vi "Read Channels.vi"(11 "HW Inline Ctrl in":T1 {"Input Channels"."Input Block Data Refs"."Data Reference" format="%.0x"; "Output Channels"."Output Block Data Refs"."Data Reference" format="%.0x"}) -> (3 "HW Inline Ctrl out":T1 {"Input Channels"."Input Block Data Refs"."Data Reference" format="%.0x"; "Output Channels"."Output Block Data Refs"."Data Reference" format="%.0x"})   [LabVIEW 2012, in "Shared Variable Custom Device.lvlib"]
doc: "Reads the values from the Input Block Data References and writes the values to the RT FIFO Read."
uses:
  Shared Variable Custom Device.lvlib
  HW Inline Ctrl.ctl
  <vilib>/NI Veristand/Custom Device API/Block Data Reference.ctl
  <vilib>/NI Veristand/Custom Device API/Data Reference.ctl
  <vilib>/NI Veristand/Custom Device API/Global Data Refs.vi
  <vilib>/NI Veristand/Custom Device API/Custom Device API.lvlib
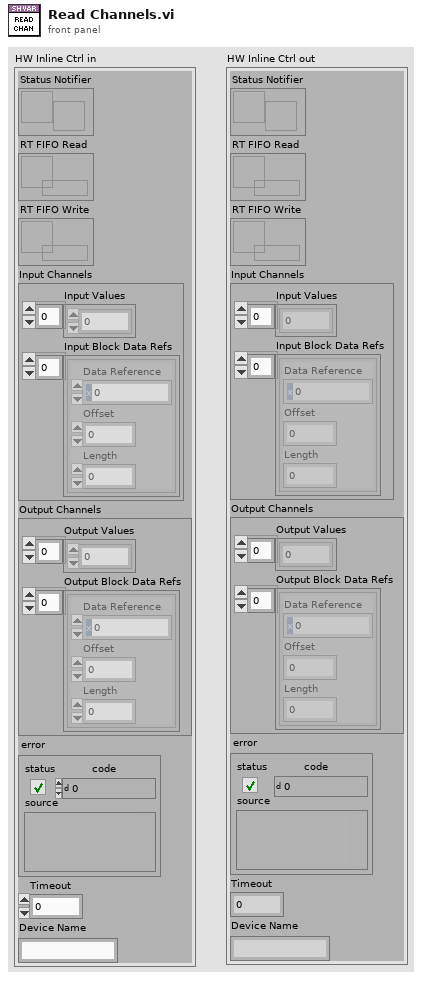
[diagram p1: front panel]
types:
  T1 = typedef "Shared Variable Custom Device.lvlib/HW Inline Ctrl.ctl" = cluster{"Status Notifier":refnum<notifier>, "RT FIFO Read":refnum<k33>, "RT FIFO Write":refnum<k33>, "Input Channels":cluster{"Input Values":dbl[], "Input Block Data Refs":T2[]}, "Output Channels":cluster{"Output Values":dbl[], "Output Block Data Refs":T2[]}, "error":errorcluster, "Timeout":i32, "Device Name":string}
  T2 = typedef "Custom Device API.lvlib/Block Data Reference.ctl" = cluster{"Data Reference":T3, "Offset":i32, "Length":i32}
  T3 = typedef "Custom Device API.lvlib/Data Reference.ctl" = i32
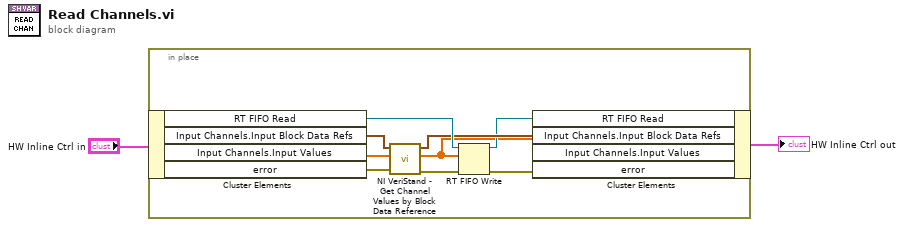
[diagram p0: block diagram]
diagram:
  n1 = in-place {
    n2 = in-place-cluster #1("HW Inline Ctrl in") -> ("RT FIFO Read"=w7:refnum<k33>, "Input Channels.Input Block Data Refs"=w10:T2[], "Input Channels.Input Values"=w9:dbl[], "error"=w11:errorcluster)
    n3 = call <vilib>:"NI VeriStand - Get Channel Values by Block Data Reference.vi"("error in (no error)"=w11, "Values Array in"=w9, "Block Data Ref"=w10) -> ("error out"=w8:errorcluster, "Values Array out"=w3:dbl[], "Block Data Ref dup"=w6:T2[])  [unwired: 6 in]
    n4 = RT FIFO Write(0:w7, 1:w3, 3:w8) -> (8:w5:refnum<k33>, 11:w4:errorcluster)  [unwired: 2 in, 2 out]
    n5 = in-place-cluster #1("RT FIFO Read"=w5, "Input Channels.Input Block Data Refs"=w6, "Input Channels.Input Values"=w3, "error"=w4) -> (→"HW Inline Ctrl out":T1)
  }
